vi "Write sound format.vi"(8 "error in (no error)":errorcluster caption="에러 입력(에러 없음)", 10 "sound format":T1={"sample rate (S/s)"=22050.0, "number of channels"=2, "bits per sample"=16} caption="사운드 포맷", 11 "WAV File 입력":refnum<class "WAV File.lvclass">) -> (0 "error out":errorcluster caption="에러 출력", 3 "WAV File 출력":refnum<class "WAV File.lvclass">)   [LabVIEW 2020, in "WAV File.lvclass"]
uses:
  WAV File.lvclass
  <vilib>/sound2/lvsound2.llb/Sound Data Format.ctl
  WAV File.lvclass/WAV File.ctl
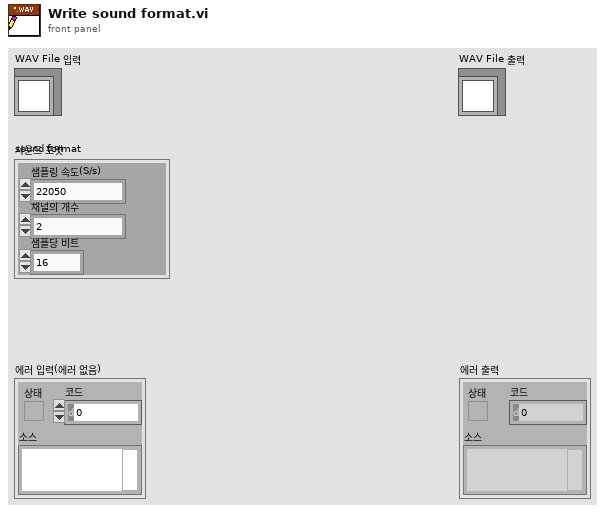
[diagram p1: front panel]
types:
  T1 = typedef "Sound Data Format.ctl" = cluster{"sample rate (S/s)":dbl, "number of channels":i32, "bits per sample":i32}
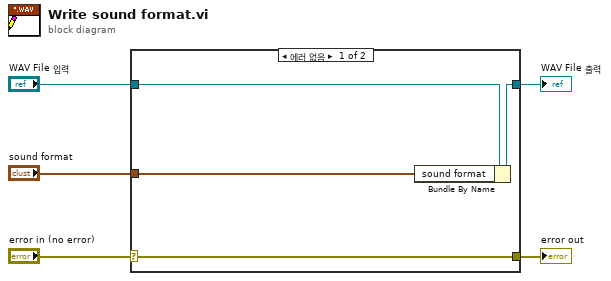
[diagram p0: block diagram]
diagram:
  n1 = case shown="에러 없음" "error in (no error)" {
    selector: "error in (no error)" -> [w9 w10]
    tunnel: [w9 w10] -> w4
    tunnel: [w7 w11] -> w2
    tunnel: "WAV File 입력" -> [w8 w11]
    tunnel: "sound format" -> [w6 _]
    frame No Error {
      n2 = Bundle By Name(cluster=w8, "sound format"=w6) -> (w7:refnum<class "WAV File.lvclass">)
    }
    frame Error {
    }
  }
  "error out" <- w4
  "WAV File 출력" <- w2
